vi "Read MFC.vi"(8 "error in (no error)":errorcluster, 10 "MFC Mode (0: Voltage)":u16(ring) items=["Voltage", "Current"], 11 "VISA resource name":refnum<visa-resource-name>) -> (0 "error out":errorcluster, 1 "MFC Supply Voltage":dbl, 2 "MFC Voltage/Current":dbl, 3 "VISA resource name out":refnum<visa-resource-name>)   [LabVIEW 2023, in "Fluke Molbox 1 Plus.lvlib"]
doc: "Reads measurements of the MFC including the voltage or current and the supply voltage. This requires the MFC to be enabled."
uses:
  Fluke Molbox 1 Plus.lvlib
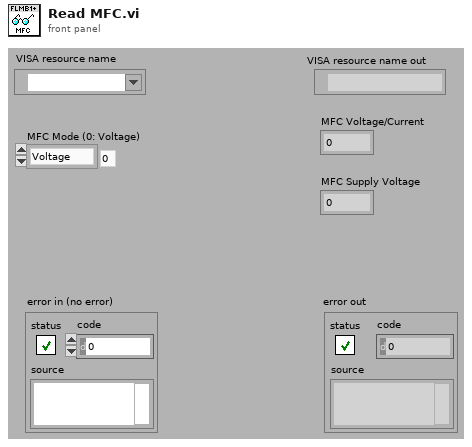
[diagram p1: front panel]
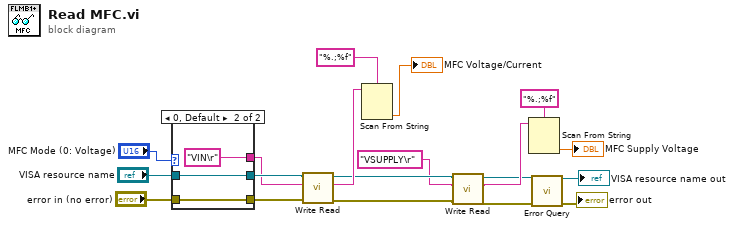
[diagram p0: block diagram]
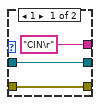
[diagram p2: hidden frame]
diagram:
  n1 = case shown="0, Default" "MFC Mode (0: Voltage)" {
    tunnel: "VISA resource name" -> [w21 w24]
    tunnel: "error in (no error)" -> [w20 w23]
    tunnel: [w21 w24] -> w12
    tunnel: [w20 w23] -> w11
    tunnel: ["CIN\r" ("write buffer") "VIN\r" ("write buffer")] -> w1
    frame 1 {
    }
    frame 0, Default {
    }
  }
  n2 = call "Write Read.vi"("error in (no error)"=w11, "Write String"=w1, "VISA resource name"=w12) -> ("error out"=w8:errorcluster, "Read Response"=w10:string, "VISA resource name out"=w9:refnum<visa-resource-name>)  [unwired: 6 in]
  n3 = Scan From String(format string="%.;%f", input string=w10) -> (output 1=→"MFC Voltage/Current":dbl)  [unwired: 3 in, 3 out]
  n4 = call "Write Read.vi"("error in (no error)"=w8, "Write String"="VSUPPLY\r" ("write buffer"), "VISA resource name"=w9) -> ("error out"=w3:errorcluster, "Read Response"=w6:string, "VISA resource name out"=w2:refnum<visa-resource-name>)  [unwired: 6 in]
  n5 = Scan From String(format string="%.;%f", input string=w6) -> (output 1=→"MFC Supply Voltage":dbl)  [unwired: 3 in, 3 out]
  n6 = call "Error Query.vi"("error in (no error)"=w3, "VISA resource name"=w2) -> ("error out"=→"error out":errorcluster, "VISA resource name out"=→"VISA resource name out":refnum<visa-resource-name>)  [unwired: 6 in, 2 out]
